vi "execute_Query.vi"(8 "error in (no error)":errorcluster, 10 "String":string, 11 "connection reference":T1) -> (0 "error out":errorcluster, 2 "Table":string[][](array[string]), 3 "connection reference 2":T1)   [LabVIEW 2017]
uses:
  <vilib>/addons/database/Connection.llb/Conn ObjectReference.ctl
  <vilib>/addons/database/Connection.llb/Conn Execute.vi
  <vilib>/addons/database/Recordset.llb/Rec Fetch Recordset Data (R).vi
  <vilib>/addons/database/Recordset.llb/Rec Destroy - Connection.vi
  <vilib>/addons/database/NI_Database_API.lvlib
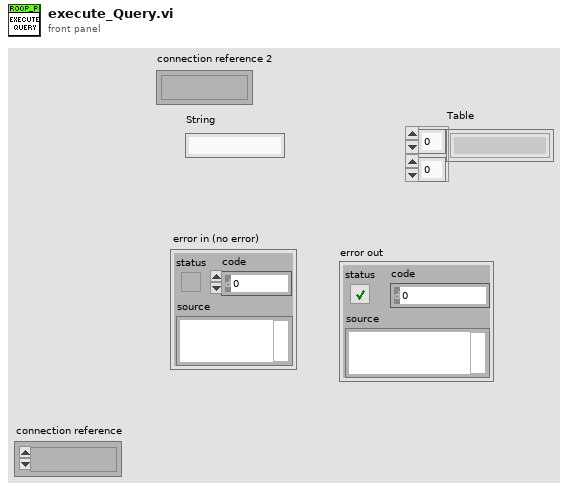
[diagram p1: front panel]
types:
  T1 = typedef "NI_Database_API.lvlib/Conn ObjectReference.ctl" = refnum<k1>
  T2 = typedef "NI_Database_API.lvlib/Rec ObjectReference.ctl" = refnum<k1>
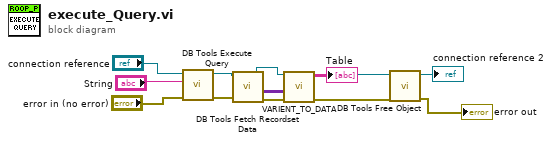
[diagram p0: block diagram]
diagram:
  n1 = call-poly <vilib>:"DB Tools Execute Query.vi"("error in (no error)"="error in (no error)", "SQL query"="String", "connection reference"="connection reference") -> ("error out"=w10:errorcluster, "recordset reference"=w5:T2)  [unwired: 5 in]
  n2 = call-poly <vilib>:"DB Tools Fetch Recordset Data.vi"("error in (no error)"=w10, "recordset reference"=w5) -> ("error out"=w9:errorcluster, "recordset data"=w11:variant[][], "recordset reference out"=w4:T2)  [unwired: 3 in]
  n3 = call "VARIENT_TO_DATA.vi"("data"=w11, "error in (no error)"=w9) -> ("Table"=→"Table":string[][], "error out"=w3:errorcluster)  [unwired: 7 in]
  n4 = call-poly <vilib>:"DB Tools Free Object.vi"("error in (no error)"=w3, "recordset reference"=w4) -> ("error out"=→"error out":errorcluster, "connection reference"=→"connection reference 2":T1)  [unwired: 8 in]
